vi "flattenToString.vi"(8 "error in (no error)":errorcluster, 11 "Task Outputs in":refnum<class "Task Outputs.lvclass">) -> (0 "error out":errorcluster, 3 "data string":string)   [LabVIEW 2017, in "Message Interface.lvlib" / "Task Outputs.lvclass"]
uses:
  Task Outputs.lvclass
  Volumes/Data/Users/benji667/Git/BuildFarm/BuildWorker/Classes/Status/Status.lvclass
  Status/Status.lvclass/Status.ctl
  Status/Read Item Name.vi
  Status/Write Item Name.vi
  Status/Status.lvclass
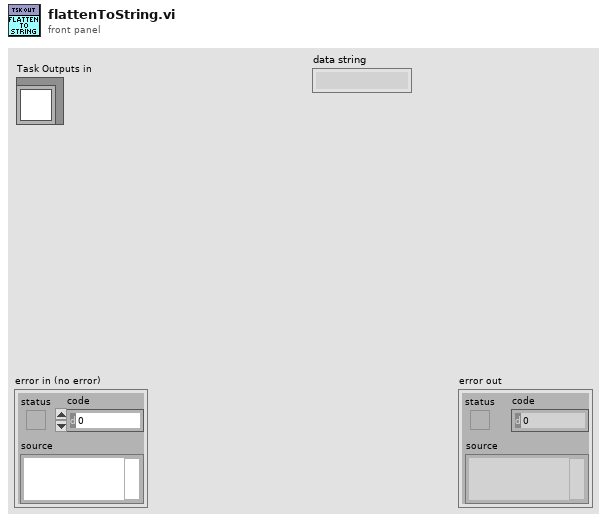
[diagram p1: front panel]
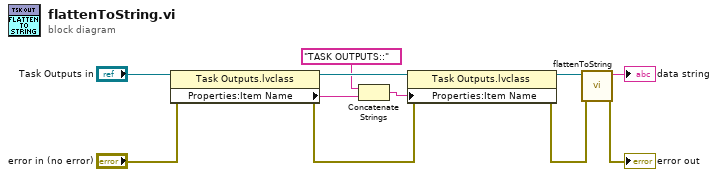
[diagram p0: block diagram]
diagram:
  n1 = property class="Task Outputs.lvclass"(reference="Task Outputs in", error in="error in (no error)") -> (reference out=w9:refnum<class "Task Outputs.lvclass">, error out=w1:errorcluster, "Properties:Item Name"=w7:string)
  n2 = Concatenate Strings("TASK OUTPUTS::" ("string"), w7) -> (w8:string)
  n3 = property class="Task Outputs.lvclass"(reference=w9, error in=w1, "Properties:Item Name"=w8) -> (reference out=w4:refnum<class "Task Outputs.lvclass">, error out=w2:errorcluster)
  n4 = call-parent "flattenToString.vi"("error in (no error)"=w2, "iMessage in"=w4) -> ("error out"=→"error out":errorcluster, "data string"=→"data string":string)  [unwired: 8 in]
